vi "calibrationElectrometer_cancelCallback_command_Start.vi"(8 "error in (no error)":errorcluster) -> (0 "error out":errorcluster, 3 "function return":i32)   [LabVIEW 2016, in "SALLV_calibrationElectrometer.lvlib"]
doc: "int calibrationElectrometer_shm_cancelCallback_command_StartLV();"
uses:
  SALLV_calibrationElectrometer.lvlib
  SALLV_calibrationElectrometer.so
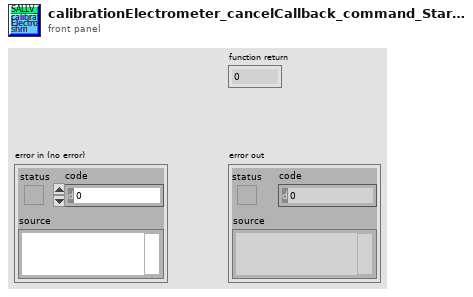
[diagram p1: front panel]
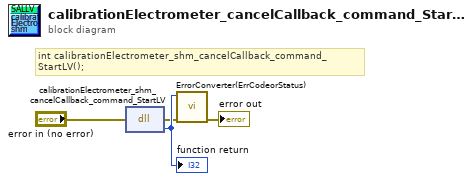
[diagram p0: block diagram]
diagram:
  # "int calibrationElectrometer_shm_cancelCallback_command_StartLV();"
  n1 = dll-call lib="home/harini/tcs/ts_SALLV_calibrationElectrometer_take2/SALLV_calibrationElectrometer.*" fn="calibrationElectrometer_shm_cancelCallback_command_StartLV"(error in="error in (no error)") -> (error out=w2:errorcluster, w4:i32)  [unwired: 2 in, 1 out]
  "function return" <- w4
  n2 = call "ErrorConverter(ErrCodeorStatus).vi"("error in (no error)"=w2, "error code"=w4) -> ("error out"=→"error out":errorcluster)  [unwired: 9 in]
